vi "Init.vi"(8 "error in (no error)":errorcluster) -> (0 "error out":errorcluster, 3 "Enclave out":refnum<class "Enclave.lvclass">)   [LabVIEW 2022 SP3, in "Enclave.lvlib" / "Enclave.lvclass"]
uses:
  Enclave.lvclass
  Enclave Event.ctl
  Element.ctl
  Tag Data.ctl
  Writer Data.ctl
  Enclave.lvclass/Enclave.ctl
  Enclave.lvlib
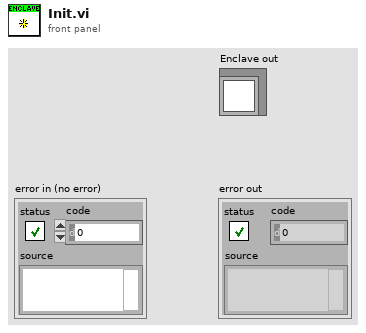
[diagram p1: front panel]
types:
  T1 = typedef "Enclave.lvlib/Writer Data.ctl" = cluster{"Queues":refnum<queue>[], "Lossy":bool, "Event":bool}
  T2 = typedef "Enclave.lvlib/Tag Data.ctl" = cluster{"Element":T3, "Sequence":u64, "Time Stamp":timestamp}
  T3 = typedef "Enclave.lvlib/Element.ctl" = dbl
  T4 = typedef "Enclave.lvlib/Enclave Event.ctl" = cluster{"Element":T3, "Closed":bool}
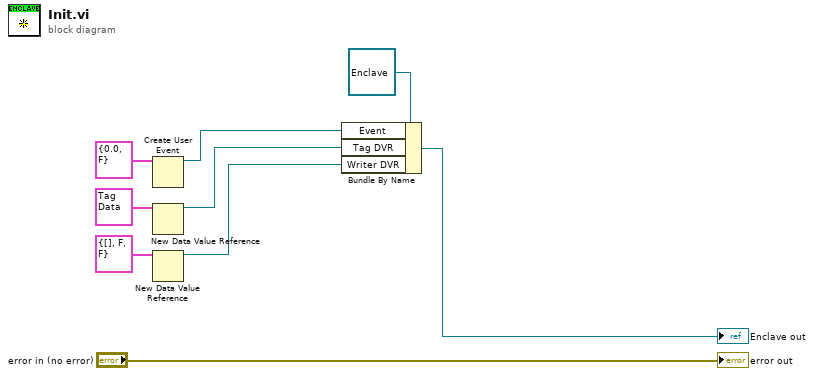
[diagram p0: block diagram]
diagram:
  n1 = Create User Event(user event datatype=T4 {"Element"=0.0, "Closed"=FALSE} ("Enclave Event")) -> (user event=w5:refnum<user-event>)  [unwired: 1 in, 1 out]
  n2 = New Data Value Reference(data value=T2 {"Element"=0.0, "Sequence"=0, "Time Stamp"=timestamp(0 s since 1904-01-01)} ("Notifier Data")) -> (data value reference=w3:refnum<data-value>)  [unwired: 1 in, 1 out]
  n3 = New Data Value Reference(data value=T1 {"Queues"=[], "Lossy"=FALSE, "Event"=FALSE} ("Writer Data")) -> (data value reference=w1:refnum<data-value>)  [unwired: 1 in, 1 out]
  n4 = Bundle By Name(cluster=refnum<class "Enclave.lvclass"> refnum ("Enclave in"), "Event"=w5, "Tag DVR"=w3, "Writer DVR"=w1) -> (→"Enclave out":refnum<class "Enclave.lvclass">)
  "error out" <- "error in (no error)"
